vi "Register Plugin.vi"(6 "timeout (ms)":i32=5000, 8 "error in":errorcluster, 10 "Register":T1, 11 "gRPC ID in":T3) -> (0 "error out":errorcluster, 2 "loader_name":string, 3 "gRPC ID out":T3)   [LabVIEW 2021, in "CIFManagerClientWrapper.lvlib"]
uses:
  CIFManagerClientWrapper.lvlib
  <vilib>/gRPC/LabVIEW gRPC Library/Shared/grpcId.ctl
  CIF_Manager_client/RPC Messages/cif_manager_RegisterPluginRequest.ctl
  CIF_Manager_client/RPC Messages/cif_common_ShortVersion.ctl
  CIF_Manager_client/CIF_Manager_client.lvlib
  <vilib>/gRPC/LabVIEW gRPC Library/grpc-lvsupport-release.lvlib
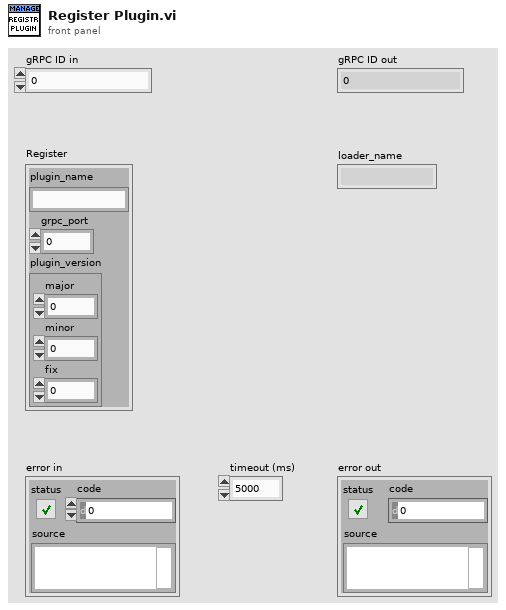
[diagram p1: front panel]
types:
  T1 = typedef "CIF_Manager_client.lvlib/cif_manager_RegisterPluginRequest.ctl" = cluster{"plugin_name":string, "grpc_port":i32, "plugin_version":T2}
  T2 = typedef "CIF_Manager_client.lvlib/cif_common_ShortVersion.ctl" = cluster{"major":u32, "minor":u32, "fix":u32}
  T3 = typedef "grpc-lvsupport-release.lvlib/grpcId.ctl" = u64
  T4 = typedef "CIF_Manager_client.lvlib/cif_manager_RegisterPluginResponse.ctl" = cluster{"loader_name":string}
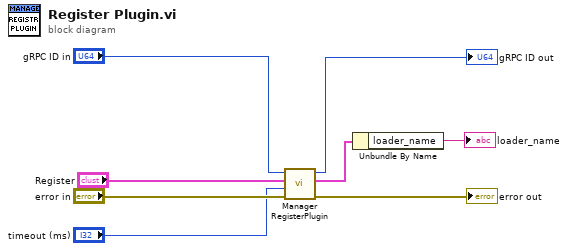
[diagram p0: block diagram]
diagram:
  n1 = call "Manager RegisterPlugin.vi"("error in"="error in", "timeout (ms)"="timeout (ms)", "Request Data"="Register", "gRPC ID"="gRPC ID in") -> ("error out"=→"error out":errorcluster, "Response Data"=w2:T4, "gRPC ID out"=→"gRPC ID out":T3)  [unwired: 5 in]
  n2 = Unbundle By Name(w2) -> ("loader_name"=→"loader_name":string)
